vi "setpoint and rotate in steps.vi"() -> ()   [LabVIEW 2016]
panel:
  in  "which axis":enum16{"move axis 1", "move axis 2"}(ring)=enum."move axis 2"
  in  "m/c temp setpoint":dbl
  in  "sp position °":dbl
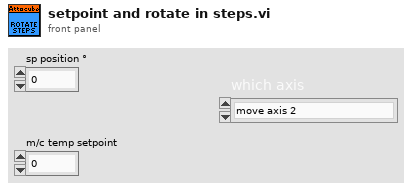
[diagram p1: front panel]
types:
  T1 = cluster{"axis 1: Current position (°)":dbl, "axis 2: Current position (°)":dbl, "axis 1: rot. count":dbl, "axis 2: rot. count":dbl, "axis 1: StepWidth":dbl, "axis 2: StepWidth":dbl, "axis 1: speed (°/s)":dbl, "axis 2: speed (°/s)":dbl, "axis 1: positioner status":cluster{"moving":bool, "stop detected":bool, "sensor error":bool, "sensor disconnected":bool}, "axis 2: positioner status":cluster{"moving":bool, "stop detected":bool, "sensor error":bool, "sensor disconnected":bool}}
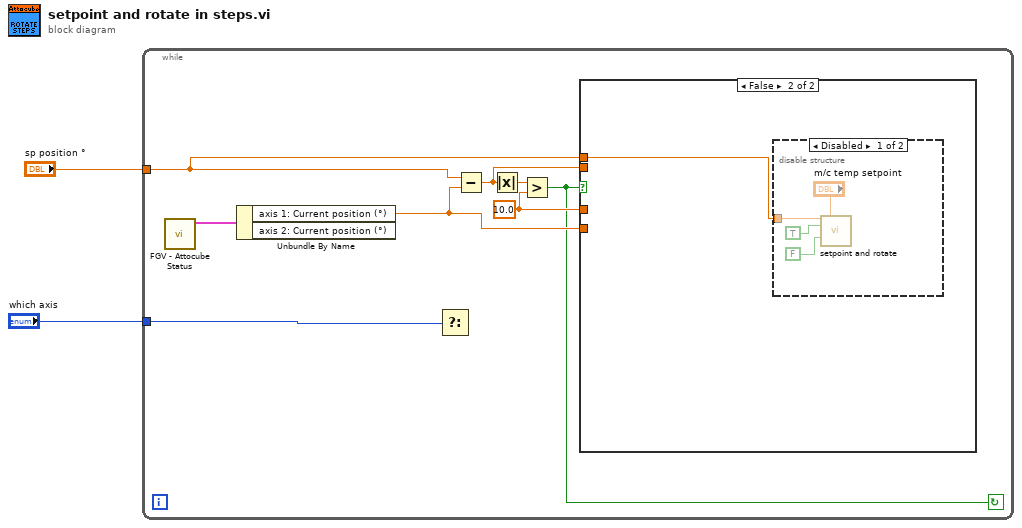
[diagram p0: block diagram]
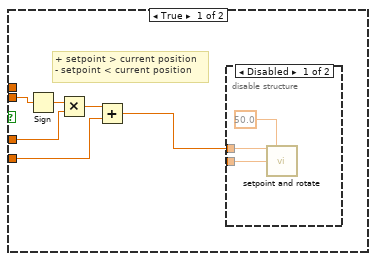
[diagram p2: hidden frame]
diagram:
  n1 = while {
    tunnel: "sp position °" -> [w9]
    tunnel: "which axis" -> [w3]
    stop <- w4 continue-if-true
    w6 = 10.0 ("y")
    n2 = call "FGV - Attocube Status.vi"() -> ("Status OUT"=w10:T1)  [unwired: 6 in, 1 out]
    n3 = Unbundle By Name(w10) -> ("axis 1: Current position (°)"=w5:dbl)  [unwired: 1 out]
    n4 = Select(s=w3) -> ()  [unwired: 2 in, 1 out]
    n5 = Subtract(x=w9, y=w5) -> (x-y=w7:dbl)
    n6 = Absolute Value(x=w7) -> (abs(x)=w8:dbl)
    n7 = Greater?(x=w8, y=w6) -> (0:w4:bool)
    n8 = case shown="False" w4 {
      tunnel: w9 -> [_ w20]
      tunnel: w7 -> [w16 _]
      tunnel: w6 -> [w11 _]
      tunnel: w5 -> [w13 _]
      frame True {
        # "+ setpoint > current position\n- setpoint < current position"
        n9 = Sign(1:w16) -> (0:w15:dbl)
        n10 = Multiply(x=w15, y=w11) -> (x*y=w14:dbl)
        n11 = Add(x=w14, y=w13) -> (x+y=w12:dbl)
        n12 = disable-structure shown="Disabled" {
          disable-tunnel: w12 -> [w19 _]
          disable-tunnel: _ -> [w18 _]
          frame Disabled {
            n13 = call "setpoint and rotate.vi"("axis 1: sp position °"=w19, "m/c temp setpoint"=50.0, "axis 2: sp position °"=w18) -> ()  [unwired: 11 in, 2 out]
          }
          frame Enabled {
          }
        }
      }
      frame False {
        n14 = disable-structure shown="Disabled" {
          disable-tunnel: w20 -> [w24 _]
          frame Disabled {
            n15 = call "setpoint and rotate.vi"("axis 1: sp position °"=w24, "m/c temp setpoint"="m/c temp setpoint", "move axis 1"=TRUE, "move axis 2"=FALSE) -> ()  [unwired: 10 in, 2 out]
          }
          frame Enabled {
          }
        }
      }
    }
  }
